vi "Mock.vi"(8 "error in":errorcluster, 10 "Message In":string, 11 "Transport Parameters In":T1={"Transport Parameters"={"Serial Communication"={"Comport"="", "No Response Timeout Ms"=10000, "Response Complete Timeout Ms"=10000, "Max Rx Length"=20, "Baud Rate"=0}, "Selected Transport"=enum."Serial Communication Port", "Initializer File Path"=path "", "Cleaner File Path"=path "", "Transporter File Path"=path ""}, "Board Capabilities"={}} {"Transport Parameters"."Serial Communication"."Baud Rate" items=["75"=75, "110"=110, "134"=134, "150"=150, "300"=300, "600"=600, "1200"=1200, "1800"=1800, "2400"=2400, "4800"=4800, "7200"=7200, "9600"=9600, "14400"=14400, "19200"=19200, "28800"=28800, "38400"=38400, "56000"=56000, "57600"=57600, "115200"=115200, "128000"=128000, "230400"=230400]}) -> (0 "error out":errorcluster, 2 "Message Out":string, 3 "Transport Parameters":T1={"Transport Parameters"={"Serial Communication"={"Comport"="", "No Response Timeout Ms"=10000, "Response Complete Timeout Ms"=10000, "Max Rx Length"=20, "Baud Rate"=0}, "Selected Transport"=enum."Serial Communication Port", "Initializer File Path"=path "", "Cleaner File Path"=path "", "Transporter File Path"=path ""}, "Board Capabilities"={}} {"Transport Parameters"."Serial Communication"."Baud Rate" items=["75"=75, "110"=110, "134"=134, "150"=150, "300"=300, "600"=600, "1200"=1200, "1800"=1800, "2400"=2400, "4800"=4800, "7200"=7200, "9600"=9600, "14400"=14400, "19200"=19200, "28800"=28800, "38400"=38400, "56000"=56000, "57600"=57600, "115200"=115200, "128000"=128000, "230400"=230400]})   [LabVIEW 2020]
doc: "Fictional transport used for testing"
uses:
  Controls/Parameters.ctl
  Controls/TransportParameters.ctl
  Controls/SupportedTransports.ctl
  Controls/FirmataPinCapabilitiesAndAnalogMapping.ctl
  Controls/FirmataPinCapability.ctl
  FirmataClient.v1/controls/FirmataPinModes.ctl
  FirmataClient.v1/FirmataClient.lvlib
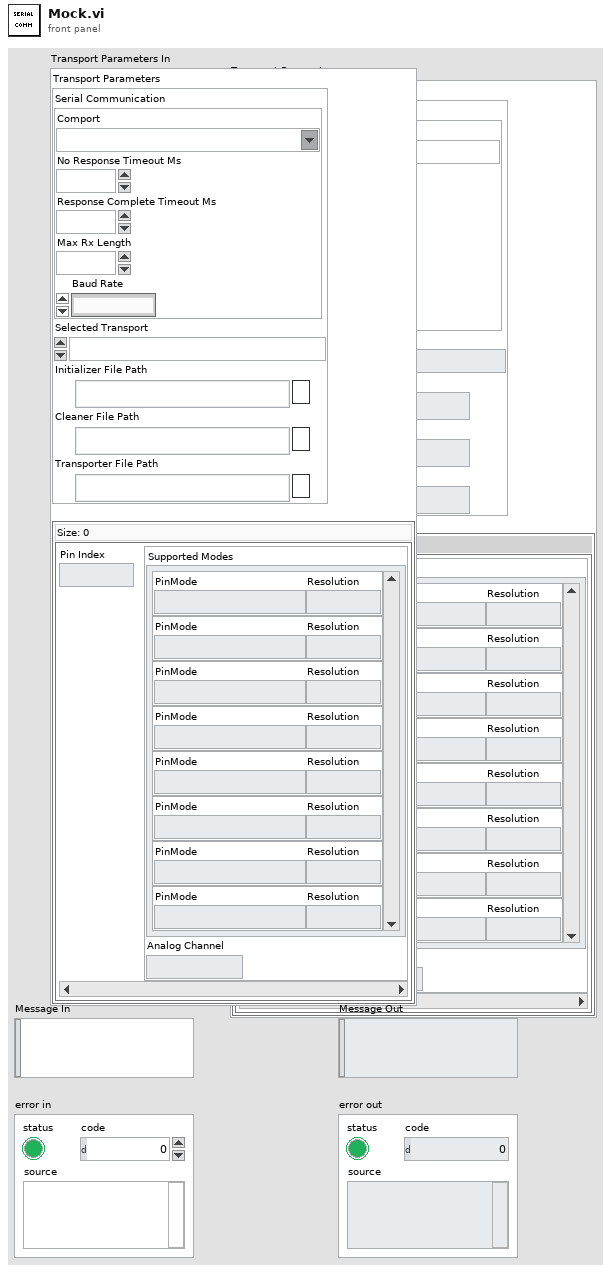
[diagram p1: front panel]
types:
  T1 = typedef "Parameters.ctl" = cluster{"Transport Parameters":T2, "Board Capabilities":map{i32, T4}}
  T2 = typedef "TransportParameters.ctl" = cluster{"Serial Communication":cluster{"Comport":refnum<visa-resource-name>, "No Response Timeout Ms":u32, "Response Complete Timeout Ms":u32, "Max Rx Length":u32, "Baud Rate":u32}, "Selected Transport":T3, "Initializer File Path":path, "Cleaner File Path":path, "Transporter File Path":path}
  T3 = typedef "SupportedTransports.ctl" = enum16{"Serial Communication Port"}
  T4 = typedef "FirmataPinCapabilitiesAndAnalogMapping.ctl" = cluster{"Supported Modes":T5[], "Analog Channel":u8}
  T5 = typedef "FirmataPinCapability.ctl" = cluster{"PinMode":T6, "Resolution":u8}
  T6 = typedef "FirmataClient.lvlib/FirmataPinModes.ctl" = enum16{"DigitalInput", "DigitalOutput", "AnalogInput", "PWM", "Servo", "Shift", "I2C", "OneWire", "Stepper", "Encoder", "Serial", "InputPullup", "Extended.SPI", "Extended.Sonar", "Extended.Tone", "Extended.DHT"}
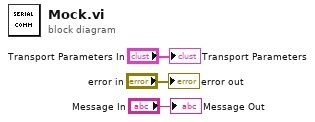
[diagram p0: block diagram]
diagram:
  "error out" <- "error in"
  "Transport Parameters" <- "Transport Parameters In"
  "Message Out" <- "Message In"
